vi "Get FPGA Reference.vi"(8 "error in (no error)":errorcluster, 10 "FPGA Reference":variant, 11 "FPGA Reference in":refnum<class "FPGA Reference.lvclass">) -> (0 "error out":errorcluster, 3 "FPGA Reference out":refnum<class "FPGA Reference.lvclass">)   [LabVIEW 2024, in "FPGA Reference.lvclass"]
uses:
  FPGA Reference.lvclass
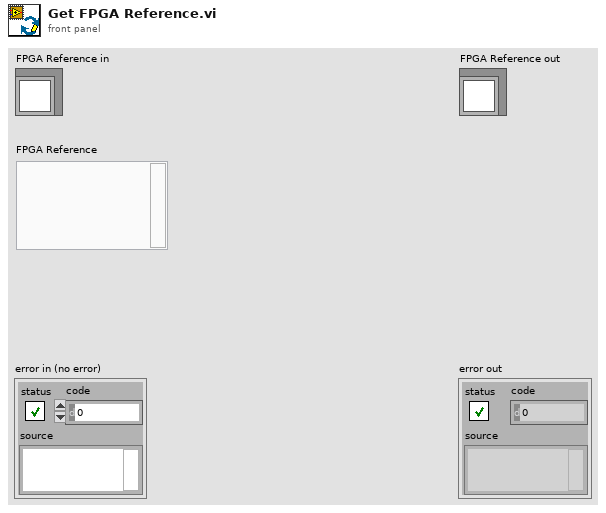
[diagram p1: front panel]
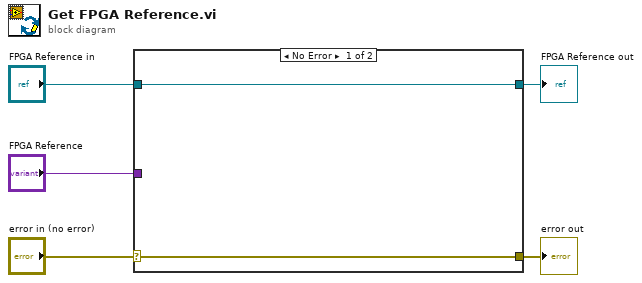
[diagram p0: block diagram]
diagram:
  n1 = case shown="No Error" "error in (no error)" {
    selector: "error in (no error)" -> [w7 w8]
    tunnel: [w7 w8] -> w4
    tunnel: [w6 w9] -> w2
    tunnel: "FPGA Reference in" -> [w6 w9]
    tunnel: "FPGA Reference" -> [_ _]
    frame No Error {
    }
    frame Error {
    }
  }
  "error out" <- w4
  "FPGA Reference out" <- w2
